vi "Teleop.vi"(10 "Match Info":T1={"Autonomous Elapsed Seconds"=0.0, "TeleOp Elapsed Seconds"=0.0, "Disabled Elapsed Seconds"=0.0, "Visited Autonomous"=FALSE, "Visited TeleOp"=FALSE, "Visited Disabled"=FALSE, "Autonomous Settings"={"Autonomous Style"=enum."Independent", "VI Refnum"=refnum}}, 11 "Call Context":T2) -> ()   [LabVIEW 2015]
doc: "This VI is called for each TeleOp packet received from the DS where the robot is not disabled. It is often used to read from the joysticks and update I/O or to update setpoints for timed control loops. It should complete and return within 20 milliseconds or it may miss DS packets."
uses:
  <vilib>/Rock Robotics/WPI/DriverStation/WPI_DriverStationDerivedRobotMode.ctl
  <vilib>/Rock Robotics/WPI/DriverStation/WPI_DriverStationMatch Info.ctl
  <vilib>/Rock Robotics/WPI/Solenoid/WPI_SolenoidValue.ctl
  <vilib>/Rock Robotics/WPI/Utilities/WPI_GetSetVariantRefNum.vi
  <vilib>/Rock Robotics/Network Tables/SD Write Boolean.vi
  <vilib>/Rock Robotics/Network Tables/SD Read Boolean.vi
  <vilib>/Rock Robotics/Network Tables/SD Read Number.vi
  <vilib>/Rock Robotics/WPI/RobotDrive/WPI_RobotDriveMecanumDrive_Cartesian.vi
  <vilib>/Rock Robotics/Network Tables/SD Write Number.vi
  <vilib>/Rock Robotics/WPI/Solenoid/WPI_SolenoidSetEnum.vi
panel:
  out "Sample Slider 0":dbl(slide) scale=0.0..5.0
  out "Sample Boolean 1":bool
  out "Sample Boolean 0":bool
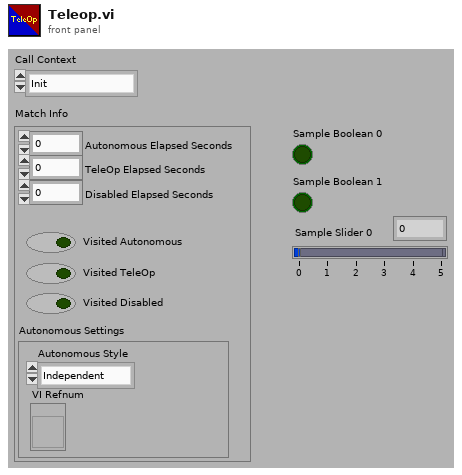
[diagram p1: front panel]
types:
  T1 = typedef "WPI_DriverStationMatch Info.ctl" = cluster{"Autonomous Elapsed Seconds":dbl, "TeleOp Elapsed Seconds":dbl, "Disabled Elapsed Seconds":dbl, "Visited Autonomous":bool, "Visited TeleOp":bool, "Visited Disabled":bool, "Autonomous Settings":cluster{"Autonomous Style":enum16{"Iterative", "Independent"}, "VI Refnum":refnum<vi>}}
  T2 = typedef "WPI_DriverStationDerivedRobotMode.ctl" = enum16{"Init", "Execute", "Stop"}
  T3 = typedef "WPI_SolenoidValue.ctl" = enum16{"Off", "On", "Forward", "Reverse"}
  T4 = typedef "WPI_JoystickDevRef.ctl" = cluster{"Device":T5}
  T5 = typedef "WPI_JoystickDeviceEnum.ctl" = enum16{"USB 0", "USB 1", "USB 2", "USB 3", "USB 4", "USB 5"}
  T6 = cluster{"Axes[0]":dbl, "Axes[1]":dbl, "Axes[2]":dbl, "Axes[3]":dbl, "Axes[4]":dbl, "Axes[5]":dbl, "Axes[6]":dbl, "Axes[7]":dbl, "Axes[8]":dbl}
  T7 = cluster{"Buttons[0]":bool, "Buttons[1]":bool, "Buttons[2]":bool, "Buttons[3]":bool, "Buttons[4]":bool, "Buttons[5]":bool, "Buttons[6]":bool, "Buttons[7]":bool, "Buttons[8]":bool}
  T8 = typedef "WPI_MotorControlDeviceRef.ctl" = cluster{"DeviceStatus":errorcluster, "Type":T9, "PWM":cluster{"PWM Channel":T10, "DeadBand":T11}, "CAN":cluster{"Device Number":u8, "Control Mode":T12, "Semaphore":T13, "Max Vout":dbl, "TalonSRX Control Mode":T14}, "Invert":bool}
  T9 = typedef "WPI_MotorControlType.ctl" = enum16{"PWM", "CAN", "CANTalonSRX"}
  T10 = typedef "FPGA_DIOPWMChannel.ctl" = enum8{"PWM 0", "PWM 1", "PWM 2", "PWM 3", "PWM 4", "PWM 5", "PWM 6", "PWM 7", "PWM 8", "PWM 9", "PWM MXP 0", "PWM MXP 1", "PWM MXP 2", "PWM MXP 3", "PWM MXP 4", "PWM MXP 5", "PWM MXP 6", "PWM MXP 7", "PWM MXP 8", "PWM MXP 9", "Invalid"}
  T11 = typedef "WPI_PWMDeadband.ctl" = cluster{"Name":string, "maxPositivePwm":i32, "minPositivePwm":i32, "centerPwm":i32, "maxNegativePwm":i32, "minNegativePwm":i32, "angularRange":u16}
  T12 = typedef "WPI_CANJaguar_ControlMode.ctl" = enum8{"Percent VBus", "Current", "Speed", "Position", "Voltage"}
  T13 = typedef "Semaphore RefNum" = refnum<k1>
  T14 = typedef "WPI_CANTalonSRX_APIControlMode.ctl" = enum8{"Percent VBus", "Speed", "Position", "Slave", "Unchanged / Invalid", "Voltage Compensation", "Current", "Motion Profile"}
  T15 = typedef "WPI_GyroDevRef.ctl" = cluster{"DevStatus":errorcluster, "Analog Channel":T16, "Offset":dbl, "Gain (VoltsPerDegree/Second)":dbl, "Gyro Type":enum16{"Analog", "XRS450"}, "Handle":i32, "SPI Bus":T17, "Device Found":bool, "Sample Rate":dbl, "Calibrate On Open":bool}
  T16 = typedef "FPGA_AIChannel.ctl" = enum8{"AI 0", "AI 1", "AI 2", "AI 3", "AI MXP 0", "AI MXP 1", "AI MXP 2", "AI MXP 3", "Invalid"}
  T17 = typedef "spi_bus.ctl" = enum16{"SPI On-Board, CS0", "SPI On-Board, CS1", "SPI On-Board, CS2", "SPI On-Board, CS3", "SPI MXP", "Invalid"}
  T18 = typedef "WPI_RobotDriveDevRef.ctl" = cluster{"DevStatus":errorcluster, "Motors[]":T8[], "Square Inputs":bool, "Max Output":dbl}
  T19 = typedef "WPI_SolenoidDevRef.ctl" = cluster{"DevStatus":errorcluster, "Pneumatics Control Module":u8, "Forward Solenoid Channel":T20, "Reverse Solenoid Channel":T20}
  T20 = typedef "WPI_SolenoidChannel.ctl" = enum8{"Solenoid 0", "Solenoid 1", "Solenoid 2", "Solenoid 3", "Solenoid 4", "Solenoid 5", "Solenoid 6", "Solenoid 7", "Invalid"}
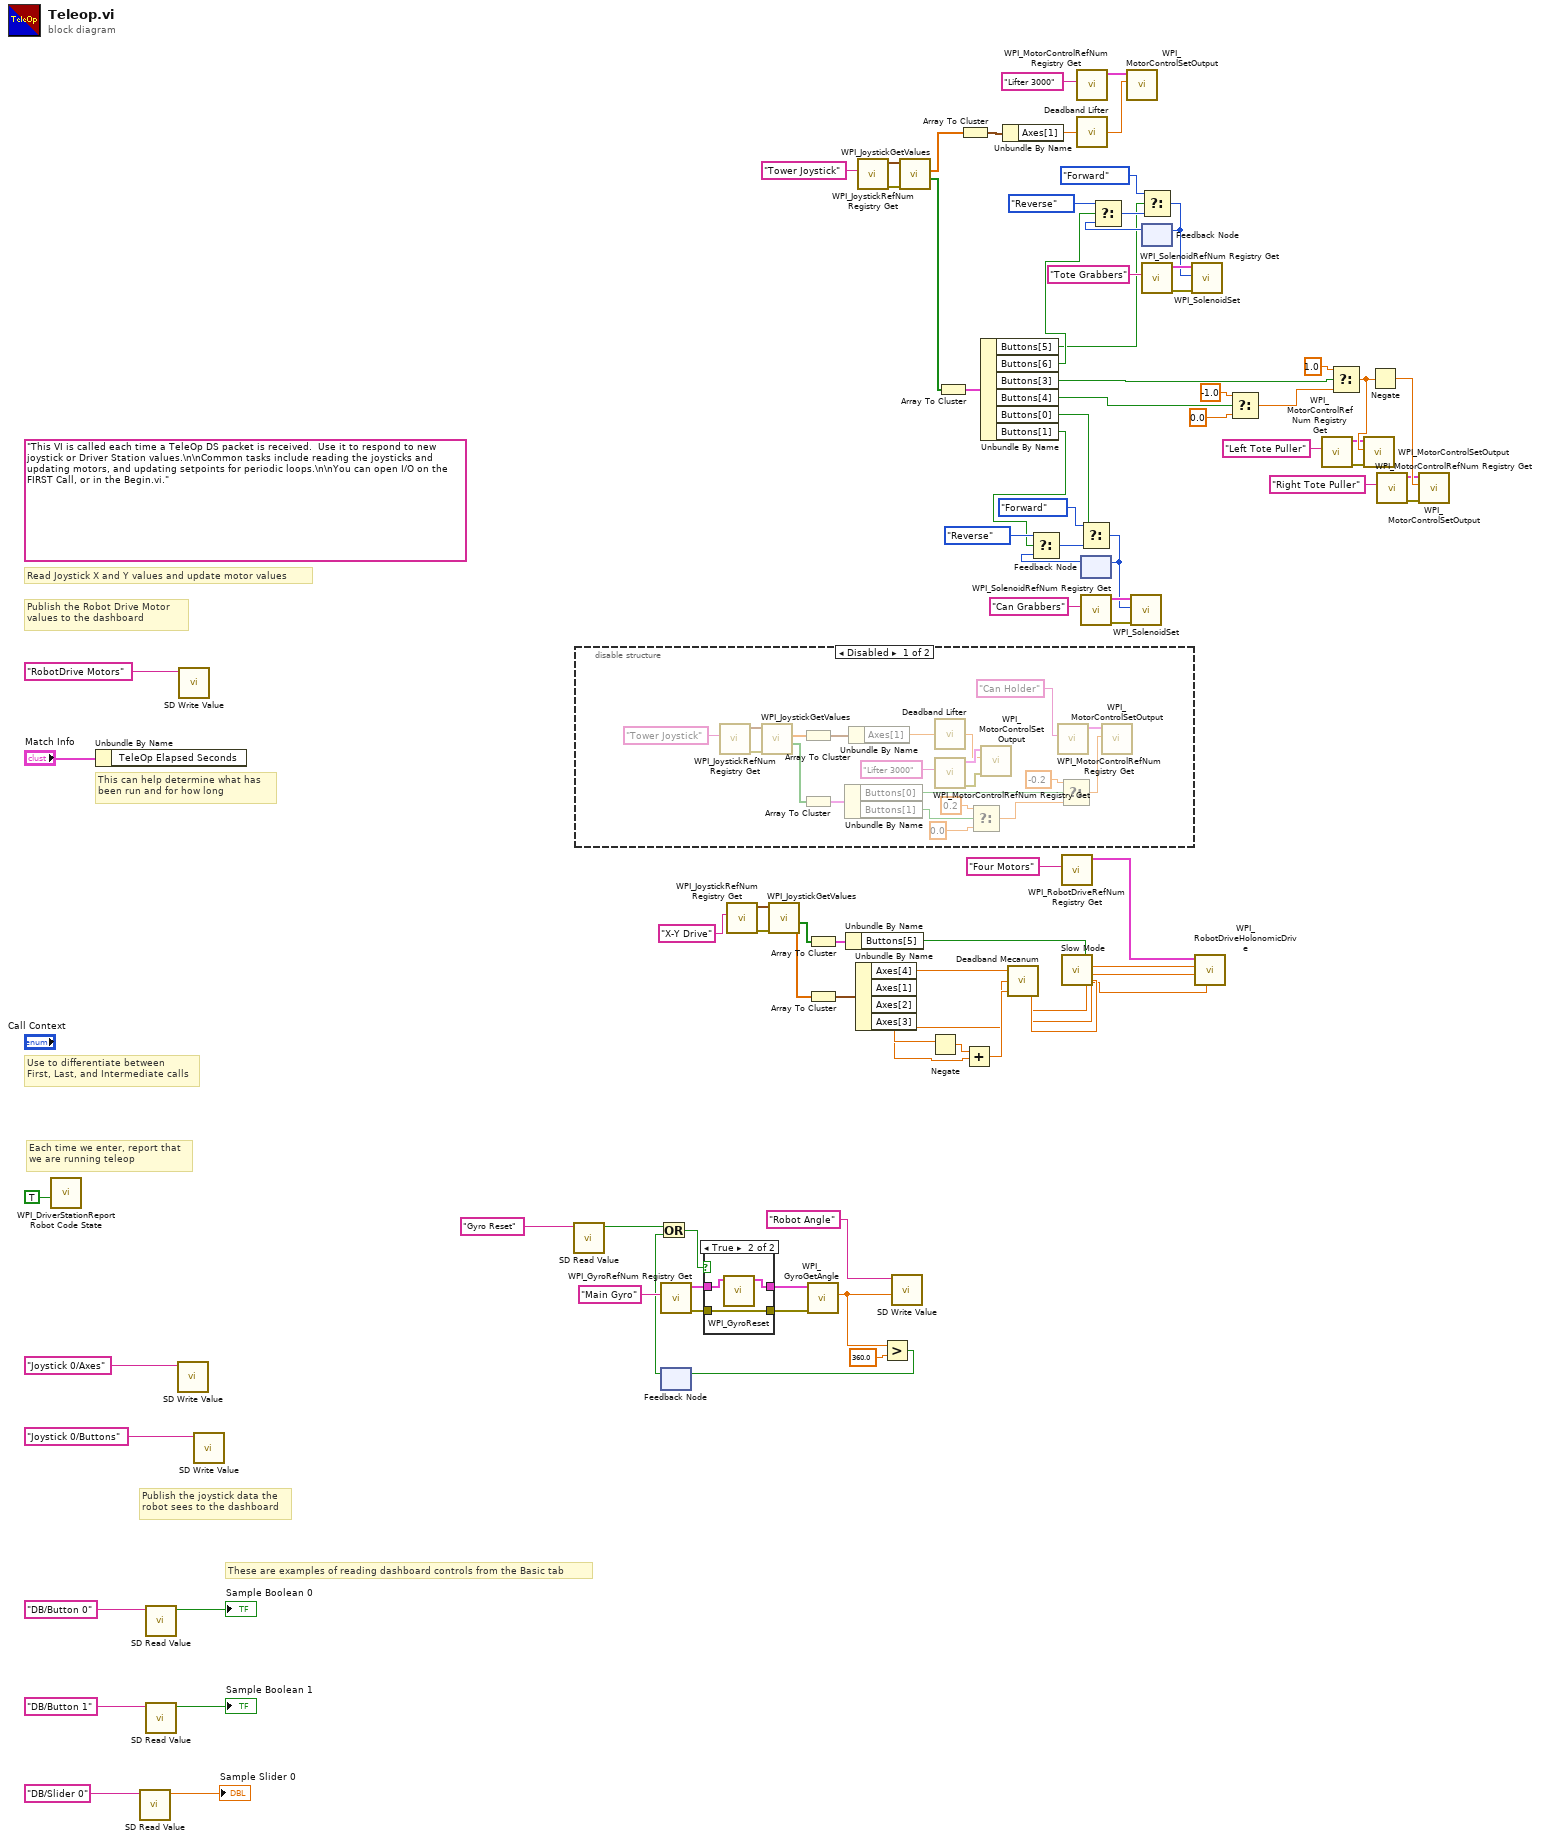
[diagram p0: block diagram]
diagram:
  (unwired) "This VI is called each time a TeleOp DS packet is received.  Use it to respond to new joystick or Driver Station values.\n\nCommon tasks include reading the joysticks and updating motors, and updating setpoints for periodic loops.\n\nYou can open I/O on the FIRST Call, or in the Begin.vi."
  # "These are examples of reading dashboard controls from the Basic tab"
  # "Publish the Robot Drive Motor\nvalues to the dashboard"
  # "Publish the joystick data the\nrobot sees to the dashboard"
  # "Each time we enter, report that\nwe are running teleop"
  # "Use to differentiate between\nFirst, Last, and Intermediate calls"
  # "This can help determine what has\nbeen run and for how long"
  # "Read Joystick X and Y values and update motor values"
  n1 = call <vilib>:"WPI_DriverStationReport Robot Code State.vi"("TeleOp"=TRUE ("Autonomous")) -> ()  [unwired: 10 in, 1 out]
  n2 = Unbundle By Name("Match Info") -> ()  [unwired: 1 out]
  n3 = call-poly <vilib>:"SD Read Value.vi"("Name"="DB/Slider 0" ("refnum name")) -> ("Numeric"=→"Sample Slider 0":dbl)  [unwired: 8 in, 2 out]
  n4 = call-poly <vilib>:"SD Read Value.vi"("Name"="DB/Button 0" ("refnum name")) -> ("Boolean"=→"Sample Boolean 0":bool)  [unwired: 8 in, 2 out]
  n5 = call-poly <vilib>:"SD Read Value.vi"("Name"="DB/Button 1" ("refnum name")) -> ("Boolean"=→"Sample Boolean 1":bool)  [unwired: 8 in, 2 out]
  n6 = call-poly <vilib>:"SD Write Value.vi"("Name"="Joystick 0/Axes") -> ()  [unwired: 9 in, 2 out]
  n7 = call-poly <vilib>:"SD Write Value.vi"("Name"="RobotDrive Motors") -> ()  [unwired: 9 in, 2 out]
  n8 = call-poly <vilib>:"SD Write Value.vi"("Name"="Joystick 0/Buttons") -> ()  [unwired: 9 in, 2 out]
  n9 = call-poly <vilib>:"SD Read Value.vi"("Name"="Gyro Reset") -> ("Boolean"=w49:bool)  [unwired: 8 in, 2 out]
  n10 = disable-structure shown="Disabled" {
    frame Disabled {
      n11 = call <vilib>:"WPI_JoystickRefNum Registry Get.vi"("refnum name"="Tower Joystick") -> ("error out"=w110:errorcluster, "JoystickDevRef"=w109:T4)  [unwired: 1 in, 8 out]
      n12 = call <vilib>:"WPI_JoystickGetValues.vi"("error in (no error)"=w110, "JoystickDevRef"=w109) -> ("Buttons"=w105:bool[], "Axes"=w107:dbl[])  [unwired: 5 in, 3 out]
      n13 = Array To Cluster(array=w107) -> (cluster=w108:T6)
      n14 = Array To Cluster(array=w105) -> (cluster=w104:T7)
      n15 = Unbundle By Name(w104) -> ("Buttons[0]"=w101:bool, "Buttons[1]"=w98:bool)
      n16 = Unbundle By Name(w108) -> ("Axes[1]"=w106:dbl)
      n17 = call "Deadband Lifter.vi"("Joystick Deadband Input"=w106) -> ("Joystick Deadband Output"=w92:dbl)
      n18 = call <vilib>:"WPI_MotorControlRefNum Registry Get.vi"("refnum name"="Lifter 3000") -> ("error out"=w94:errorcluster, "MotorControlDevRef"=w93:T8)  [unwired: 9 in]
      n19 = Select(t=0.2, s=w98, f=0.0) -> (s? t:f=w95:dbl)
      n20 = call <vilib>:"WPI_MotorControlSetOutput.vi"("error in (no error)"=w94, "Output"=w92, "MotorControlDevRef"=w93) -> ()  [unwired: 6 in, 3 out]
      n21 = call <vilib>:"WPI_MotorControlRefNum Registry Get.vi"("refnum name"="Can Holder") -> ("MotorControlDevRef"=w102:T8)  [unwired: 9 in, 1 out]
      n22 = Select(t=-0.2, s=w101, f=w95) -> (s? t:f=w100:dbl)
      n23 = call <vilib>:"WPI_MotorControlSetOutput.vi"("Output"=w100, "MotorControlDevRef"=w102) -> ()  [unwired: 7 in, 3 out]
    }
    frame Enabled {
    }
  }
  n24 = call <vilib>:"WPI_GyroRefNum Registry Get.vi"("refnum name"="Main Gyro") -> ("error out"=w47:errorcluster, "GyroDevRef"=w56:T15)  [unwired: 9 in]
  n25 = feedback #1() -> (w51:bool)  [unwired: 1 in]
  n26 = Or(x=w49, y=w51) -> (x .or. y?=w50:bool)
  n27 = case shown="True" w50 {
    tunnel: w56 -> [w114 w117]
    tunnel: [w114 w116] -> w55
    tunnel: w47 -> [w113 w115]
    tunnel: [w113 w115] -> w46
    frame False {
    }
    frame True {
      n28 = call <vilib>:"WPI_GyroReset.vi"("GyroDevRef"=w117) -> ("GyroDevRef"=w116:T15)  [unwired: 9 in, 1 out]
    }
  }
  n29 = call <vilib>:"WPI_JoystickRefNum Registry Get.vi"("refnum name"="X-Y Drive") -> ("error out"=w77:errorcluster, "JoystickDevRef"=w76:T4)  [unwired: 1 in, 8 out]
  n30 = call <vilib>:"WPI_JoystickGetValues.vi"("error in (no error)"=w77, "JoystickDevRef"=w76) -> ("Buttons"=w67:bool[], "Axes"=w75:dbl[])  [unwired: 5 in, 3 out]
  n31 = Array To Cluster(array=w67) -> (cluster=w66:T7)
  n32 = Array To Cluster(array=w75) -> (cluster=w74:T6)
  n33 = call <vilib>:"WPI_GyroGetAngle.vi"("error in"=w46, "GyroDevRef"=w55) -> ("Angle"=w54:dbl)  [unwired: 5 in, 4 out]
  n34 = Unbundle By Name(w66) -> ("Buttons[5]"=w57:bool)
  n35 = Unbundle By Name(w74) -> ("Axes[4]"=w68:dbl, "Axes[1]"=w69:dbl, "Axes[2]"=w73:dbl, "Axes[3]"=w71:dbl)
  n36 = call <vilib>:"WPI_JoystickRefNum Registry Get.vi"("refnum name"="Tower Joystick") -> ("error out"=w44:errorcluster, "JoystickDevRef"=w45:T4)  [unwired: 1 in, 8 out]
  n37 = Greater?(x=w54, y=360.0) -> (0:w53:bool)
  n38 = feedback-in #1(w53) -> ()
  n39 = call-poly <vilib>:"SD Write Value.vi"("Numeric"=w54, "Name"="Robot Angle") -> ()  [unwired: 8 in, 2 out]
  n40 = call <vilib>:"WPI_JoystickGetValues.vi"("error in (no error)"=w44, "JoystickDevRef"=w45) -> ("Buttons"=w42:bool[], "Axes"=w40:dbl[])  [unwired: 5 in, 3 out]
  n41 = Negate(x=w73) -> (-x=w72:dbl)
  n42 = Array To Cluster(array=w42) -> (cluster=w41:T7)
  n43 = Array To Cluster(array=w40) -> (cluster=w39:T6)
  n44 = Add(x=w72, y=w71) -> (x+y=w70:dbl)
  n45 = Unbundle By Name(w41) -> ("Buttons[5]"=w25:bool, "Buttons[6]"=w34:bool, "Buttons[3]"=w11:bool, "Buttons[4]"=w12:bool, "Buttons[0]"=w1:bool, "Buttons[1]"=w7:bool)
  n46 = Unbundle By Name(w39) -> ("Axes[1]"=w38:dbl)
  n47 = call "Deadband Mecanum.vi"("Axes 2 and 3 Deadband Input"=w70, "Axes 1 Deadband Input"=w69, "Axes 4 Deadband Input"=w68) -> ("Axes 2 and 3 Deadband Output"=w63:dbl, "Axes 1 Deadband Output"=w62:dbl, "Axes 4 Deadband Output"=w61:dbl)
  n48 = call <vilib>:"WPI_RobotDriveRefNum Registry Get.vi"("refnum name"="Four Motors") -> ("RobotDriveDevRef"=w78:T18)  [unwired: 1 in, 9 out]
  n49 = call "Slow Mode.vi"("Axes 4 Input"=w61, "Axes 1 Input"=w62, "Rotations Input"=w63, "Boolean"=w57) -> ("Axes 4 Output"=w58:dbl, "Axes 1 Output"=w59:dbl, "Rotations Output"=w60:dbl)
  n50 = call <vilib>:"WPI_MotorControlRefNum Registry Get.vi"("refnum name"="Lifter 3000") -> ("MotorControlDevRef"=w37:T8)  [unwired: 9 in, 1 out]
  n51 = call "Deadband Lifter.vi"("Joystick Deadband Input"=w38) -> ("Joystick Deadband Output"=w35:dbl)
  n52 = feedback #2() -> (w2:T3)  [unwired: 1 in]
  n53 = Select(t=WPI_SolenoidValue."Reverse" ("Value"), s=w7, f=w2) -> (s? t:f=w9:T3)
  n54 = Select(t=WPI_SolenoidValue."Forward" ("Value"), s=w1, f=w9) -> (s? t:f=w3:T3)
  n55 = feedback-in #2(w3) -> ()
  n56 = call <vilib>:"WPI_SolenoidRefNum Registry Get.vi"("refnum name"="Can Grabbers") -> ("error out"=w5:errorcluster, "SolenoidDevRef"=w6:T19)  [unwired: 9 in]
  n57 = call <vilib>:"WPI_MotorControlSetOutput.vi"("Output"=w35, "MotorControlDevRef"=w37) -> ()  [unwired: 7 in, 3 out]
  n58 = call-poly <vilib>:"WPI_SolenoidSet.vi"("error in (no error)"=w5, "Value"=w3, "SolenoidDevRef"=w6) -> ()  [unwired: 7 in, 2 out]
  n59 = feedback #3() -> (w26:T3)  [unwired: 1 in]
  n60 = Select(t=WPI_SolenoidValue."Reverse" ("Value"), s=w34, f=w26) -> (s? t:f=w29:T3)
  n61 = Select(t=WPI_SolenoidValue."Forward" ("Value"), s=w25, f=w29) -> (s? t:f=w27:T3)
  n62 = feedback-in #3(w27) -> ()
  n63 = call <vilib>:"WPI_SolenoidRefNum Registry Get.vi"("refnum name"="Tote Grabbers") -> ("error out"=w32:errorcluster, "SolenoidDevRef"=w33:T19)  [unwired: 9 in]
  n64 = call-poly <vilib>:"WPI_SolenoidSet.vi"("error in (no error)"=w32, "Value"=w27, "SolenoidDevRef"=w33) -> ()  [unwired: 7 in, 2 out]
  n65 = call-poly <vilib>:"WPI_RobotDriveHolonomicDrive.vi"("Rotation"=w60, "Y"=w59, "X"=w58, "RobotDriveDevRef"=w78) -> ()  [unwired: 5 in, 3 out]
  n66 = Select(t=-1.0, s=w12, f=0.0) -> (s? t:f=w22:dbl)
  n67 = call <vilib>:"WPI_MotorControlRefNum Registry Get.vi"("refnum name"="Left Tote Puller") -> ("error out"=w15:errorcluster, "MotorControlDevRef"=w16:T8)  [unwired: 9 in]
  n68 = Select(t=1.0, s=w11, f=w22) -> (s? t:f=w23:dbl)
  n69 = call <vilib>:"WPI_MotorControlSetOutput.vi"("error in (no error)"=w15, "Output"=w23, "MotorControlDevRef"=w16) -> ()  [unwired: 6 in, 3 out]
  n70 = Negate(x=w23) -> (-x=w24:dbl)
  n71 = call <vilib>:"WPI_MotorControlRefNum Registry Get.vi"("refnum name"="Right Tote Puller") -> ("error out"=w17:errorcluster, "MotorControlDevRef"=w18:T8)  [unwired: 9 in]
  n72 = call <vilib>:"WPI_MotorControlSetOutput.vi"("error in (no error)"=w17, "Output"=w24, "MotorControlDevRef"=w18) -> ()  [unwired: 6 in, 3 out]
